vi "UpdateCalendar.vi"(8 "error in (no error)":errorcluster, 11 "Calendar in":refnum<class "Calendar.lvclass">) -> (0 "error out":errorcluster, 3 "Calendar out":refnum<class "Calendar.lvclass">)   [LabVIEW 2015, in "Calendar.lvclass"]
uses:
  Calendar.lvclass
  <vilib>/Utility/miscctls.llb/LVRowAndColumnTypeDef.ctl
  <vilib>/Utility/miscctls.llb/LVBoundsTypeDef.ctl
  Calendar.lvclass/Calendar.ctl
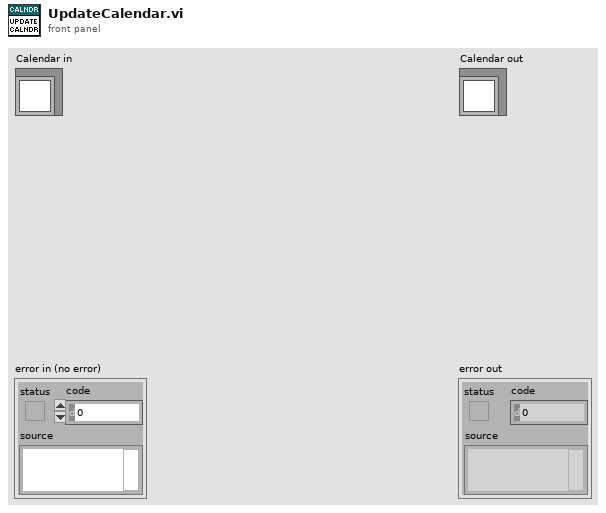
[diagram p1: front panel]
types:
  T1 = typedef "LVBoundsTypeDef.ctl" = cluster{"Width":u32, "Height":u32}
  T2 = typedef "LVRowAndColumnTypeDef.ctl" = cluster{"Row":i32, "Column":i32}
  T3 = typedef "Calendar.lvclass/State Data.ctl" = cluster{"Current Date":timestamp, "First Day of Week":T4, "Color":cluster{"Selector Background":u32, "Selector Text":u32, "Days of Week Background":u32, "Days of Week Text":u32, "Calendar Background":u32, "Calendar Text":u32, "Calendar Selection Background":u32, "Calendar Selection Text":u32}, "Visible":cluster{"Today Selector Visible":bool, "Month-Year Selector Visible":bool}}
  T4 = typedef "Calendar.lvclass/DaysOfWeek.ctl" = enum16{"Sunday", "Monday", "Tuesday", "Wednesday", "Thursday", "Friday", "Saturday"}
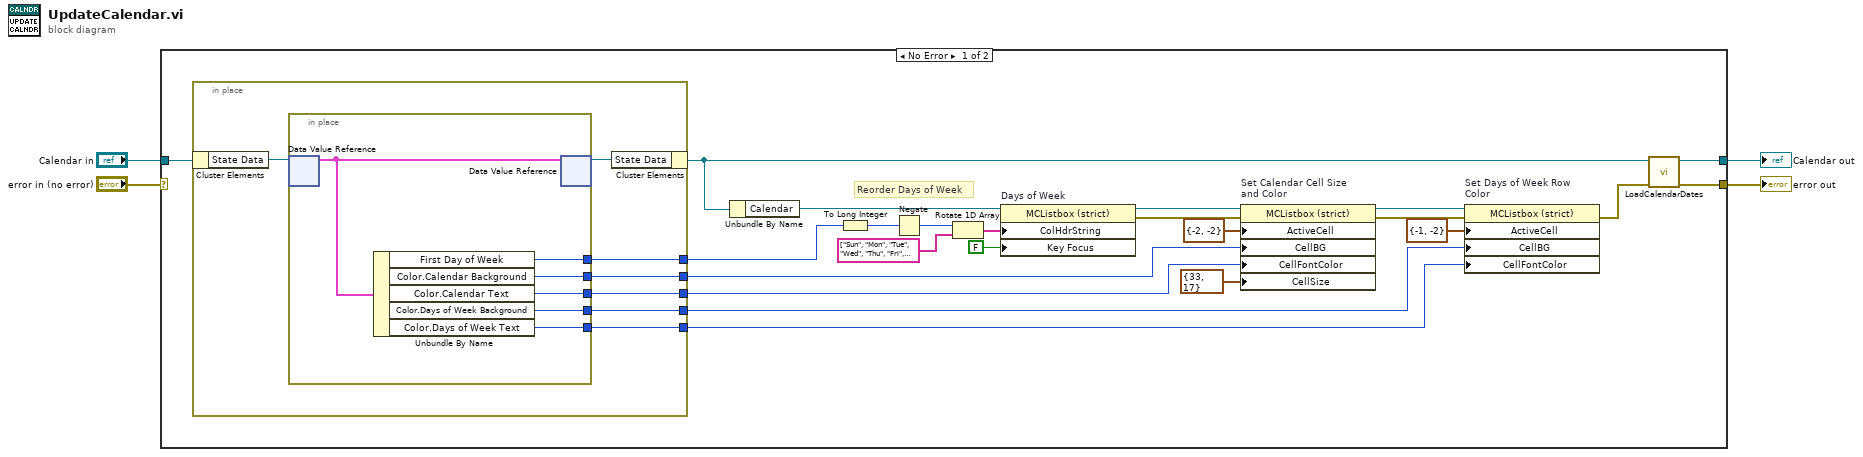
[diagram p0: block diagram]
diagram:
  n1 = case shown="No Error" "error in (no error)" {
    selector: "error in (no error)" -> [_ w42]
    tunnel: [w25 w42] -> w3
    tunnel: [w26 w41] -> w1
    tunnel: "Calendar in" -> [w27 w41]
    frame No Error {
      # "Reorder Days of Week"
      n2 = in-place {
        in-place-border: [w32] -> w10
        in-place-border: [w31] -> w9
        in-place-border: [w30] -> w8
        in-place-border: [w29] -> w7
        in-place-border: [w28] -> w5
        n3 = in-place-cluster #1(w27) -> ("State Data"=w34:refnum<data-value>)
        n4 = in-place {
          in-place-border: [w39] -> w32
          in-place-border: [w38] -> w31
          in-place-border: [w37] -> w30
          in-place-border: [w36] -> w29
          in-place-border: [w35] -> w28
          n5 = in-place-dvr #2(w34) -> (w40:T3)  [unwired: 1 out]
          n6 = Unbundle By Name(w40) -> ("First Day of Week"=w39:T4, "Color.Calendar Background"=w38:u32, "Color.Calendar Text"=w37:u32, "Color.Days of Week Background"=w36:u32, "Color.Days of Week Text"=w35:u32)
          n7 = in-place-dvr #2(w40) -> (w33:refnum<data-value>)  [unwired: 1 out]
        }
        n8 = in-place-cluster #1("State Data"=w33) -> (w24:refnum<class "Calendar.lvclass">)
      }
      n9 = Unbundle By Name(w24) -> ("Calendar"=w11:refnum<vi>)
      n10 = To Long Integer(number=w10) -> (32bit integer=w13:i32)
      n11 = Negate(x=w13) -> (-x=w14:i32)
      n12 = Rotate 1D Array(1:string[] ["Sun", "Mon", "Tue", "Wed", "Thu", "Fri", "Sat"] ("wdnames"), 2:w14) -> (0:w16:string[])
      n13 = property on="Days of Week" class="MCListbox (strict)"(reference=w11, "ColHdrString"=w16, "Key Focus"=FALSE) -> (reference out=w17:refnum<vi>, error out=w21:errorcluster)  [unwired: 1 in]
      n14 = property on="Set Calendar Cell Size\nand Color" class="MCListbox (strict)"(reference=w17, error in=w21, "ActiveCell"=T2 {"Row"=-2, "Column"=-2} ("Active Cell:Active Cell"), "CellBG"=w9, "CellFontColor"=w8, "CellSize"=T1 {"Width"=33, "Height"=17} ("Active Cell:Cell Size")) -> (reference out=w19:refnum<vi>, error out=w22:errorcluster)
      n15 = property on="Set Days of Week Row \nColor" class="MCListbox (strict)"(reference=w19, error in=w22, "ActiveCell"=T2 {"Row"=-1, "Column"=-2} ("Active Cell:Active Cell"), "CellBG"=w7, "CellFontColor"=w5) -> (error out=w6:errorcluster)  [unwired: 1 out]
      n16 = call "LoadCalendarDates.vi"("error in (no error)"=w6, "Calendar in"=w24) -> ("error out"=w25:errorcluster, "Calendar (dup)"=w26:refnum<class "Calendar.lvclass">)  [unwired: 8 in]
    }
    frame Error {
    }
  }
  "error out" <- w3
  "Calendar out" <- w1
